vi "Trigger.vi"(10 "Data In":dbl[](array[numeric]), 11 "Trigger Set":dbl) -> ()   [LabVIEW 2012]
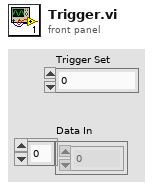
[diagram p1: front panel]
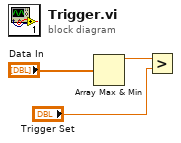
[diagram p0: block diagram]
diagram:
  n1 = Array Max & Min(array="Data In") -> (max value=w2:dbl)  [unwired: 3 out]
  n2 = Greater?(x=w2, y="Trigger Set") -> ()  [unwired: 1 out]
